vi "New Progress Window.vi"(8 "error in (no error)":errorcluster, 10 "Initial Message":string, 11 "Window Title":string="Progress Window") -> (0 "error out":errorcluster, 2 "DVRs":T1, 3 "VI refnum":refnum<vi>)   [LabVIEW 2017, in "Build Automation.lvlib"]
uses:
  Build Automation.lvlib
  Progress Window.vi
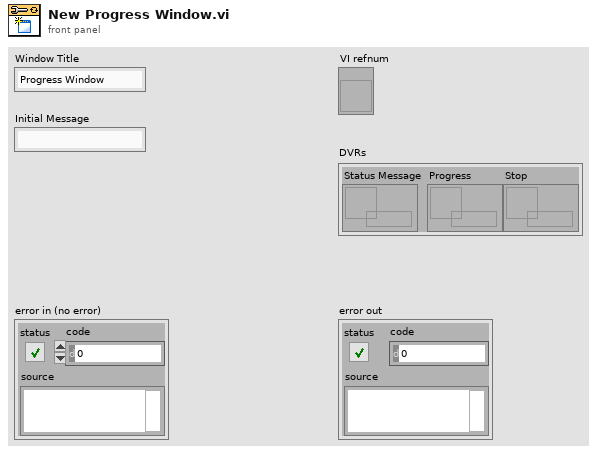
[diagram p1: front panel]
types:
  T1 = cluster{"Status Message":refnum<data-value>, "Progress":refnum<data-value>, "Stop":refnum<data-value>}
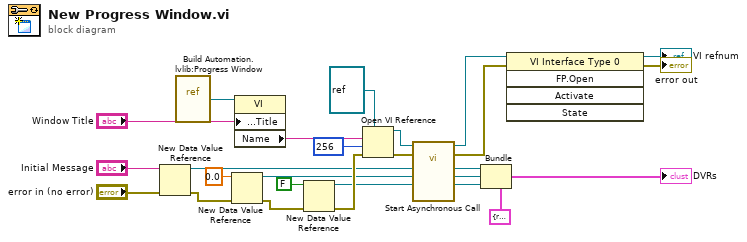
[diagram p0: block diagram]
diagram:
  n1 = New Data Value Reference(data value="Initial Message", error in="error in (no error)") -> (data value reference=w11:refnum<data-value>, error out=w21:errorcluster)
  n2 = vi-ref "Build Automation.lvlib:Progress Window.vi"() -> (w4:refnum<vi>)
  n3 = New Data Value Reference(data value=0.0, error in=w21) -> (data value reference=w10:refnum<data-value>, error out=w22:errorcluster)
  n4 = property class="VI"(reference=w4, "Front Panel.Title"="Window Title") -> ("Name"=w3:string)  [unwired: 1 in, 2 out]
  n5 = New Data Value Reference(data value=FALSE, error in=w22) -> (data value reference=w12:refnum<data-value>, error out=w15:errorcluster)
  n6 = Open VI Reference(type specifier VI Refnum (for type only)=refnum<vi> refnum, vi path=w3, options=256, error in (no error)=w15) -> (vi reference=w17:refnum<vi>, error out=w18:errorcluster)  [unwired: 2 in]
  n7 = call-by-ref "Start Asynchronous Call"(reference=w17, error in=w18, "Stop"=w12, "Progress"=w10, "Status String"=w11) -> (reference out=w8:refnum<vi>, error out=w6:errorcluster)  [unwired: 9 in]
  n8 = Bundle(cluster=T1 {"Status Message"=refnum, "Progress"=refnum, "Stop"=refnum} ("DVRs"), "Status Message"=w11, "Progress"=w10, "Stop"=w12) -> (→"DVRs":T1)
  n9 = invoke class="VI Interface Type 0" method="FP.Open"(reference=w8, error in=w6) -> (reference out=→"VI refnum":refnum<vi>, error out=→"error out":errorcluster)  [unwired: 3 in, 3 out]
